vi "Climb.vi"(9 "Abort":bool=TRUE, 11 "Start Climb Up":bool=TRUE) -> ()   [LabVIEW 2012]
uses:
  ClimberLimitSwitches.ctl
panel:
  in  "State Overide":i32
  in  "Overide State":bool
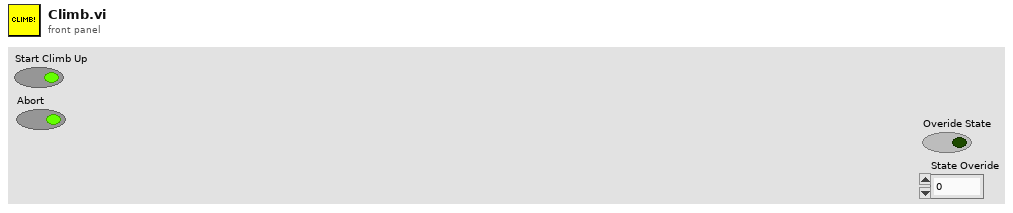
[diagram p1: front panel]
types:
  T1 = typedef "ClimberLimitSwitches.ctl" = enum16{"Off", "Bottom", "1", "2", "3", "4", "Top"}
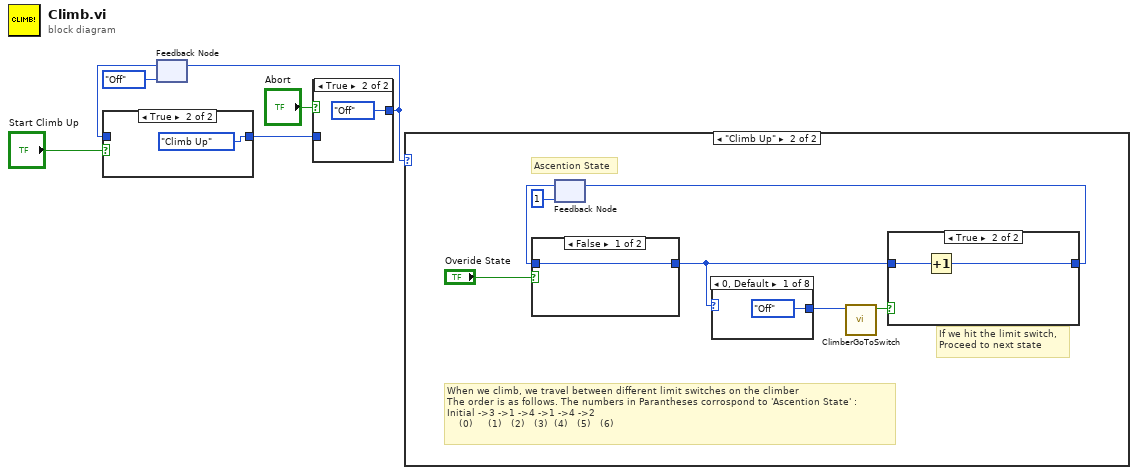
[diagram p0: block diagram]
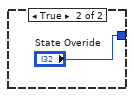
[diagram p3: hidden frame]
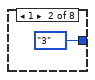
[diagram p4: hidden frame]
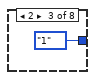
[diagram p5: hidden frame]
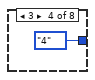
[diagram p6: hidden frame]
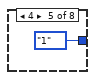
[diagram p7: hidden frame]
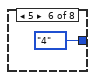
[diagram p8: hidden frame]
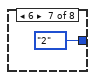
[diagram p9: hidden frame]
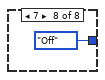
[diagram p10: hidden frame]
diagram:
  n1 = feedback #1(enum16{"Off", "Climb Up", "Climb Down"}."Off") -> (w1:enum16{"Off", "Climb Up", "Climb Down"})
  n2 = case shown="True" "Start Climb Up" {
    tunnel: w1 -> [w7 _]
    tunnel: [w7 enum16{"Off", "Climb Up", "Climb Down"}."Climb Up"] -> w3
    frame False {
    }
    frame True {
    }
  }
  n3 = case shown="True" "Abort" {
    tunnel: w3 -> [w9 _]
    tunnel: [w9 enum16{"Off", "Climb Up", "Climb Down"}."Off"] -> w2
    frame False {
    }
    frame True {
    }
  }
  n4 = feedback-in #1(w2) -> ()
  n5 = case shown="\"Climb Up\"" w2 {
    frame "Off", Default {
    }
    frame "Climb Up" {
      # "When we climb, we travel between different limit switches on the climber\nThe order is as follows. The numbers in Parantheses corrospond to 'Ascention State' :\nInitial ->3 ->1 ->4 ->1 ->4 ->2 \n    (0)     (1)   (2)   (3)  (4)   (5)   (6)"
      # "If we hit the limit switch,\nProceed to next state"
      # "Ascention State"
      n6 = feedback #2(1) -> (w12:i32)
      n7 = case shown="False" "Overide State" {
        tunnel: [w18 "State Overide"] -> w11
        tunnel: w12 -> [w18 _]
        frame False {
        }
        frame True {
        }
      }
      n8 = case shown="0, Default" w11 {
        tunnel: [ClimberLimitSwitches."Off" ("TargetSwitch") ClimberLimitSwitches."3" ("TargetSwitch") ClimberLimitSwitches."1" ("TargetSwitch") ClimberLimitSwitches."4" ("TargetSwitch") ClimberLimitSwitches."1" ("TargetSwitch") ClimberLimitSwitches."4" ("TargetSwitch") ClimberLimitSwitches."2" ("TargetSwitch") ClimberLimitSwitches."Off" ("TargetSwitch")] -> w15
        frame 0, Default {
        }
        frame 1 {
        }
        frame 2 {
        }
        frame 3 {
        }
        frame 4 {
        }
        frame 5 {
        }
        frame 6 {
        }
        frame 7 {
        }
      }
      n9 = call "ClimberGoToSwitch.vi"("TargetSwitch"=w15) -> ("Done"=w14:bool)  [unwired: 10 in]
      n10 = case shown="True" w14 {
        tunnel: w11 -> [w28 w30]
        tunnel: [w28 w29] -> w17
        frame False {
        }
        frame True {
          n11 = Increment(x=w30) -> (x+1=w29:i32)
        }
      }
      n12 = feedback-in #2(w17) -> ()
    }
  }
